vi "HandleIncomingPacket.vi"(8 "error in (no error)":errorcluster, 11 "ControlPacket in":refnum<class "ControlPacket.lvclass">) -> (0 "error out":errorcluster, 3 "ControlPacket out":refnum<class "ControlPacket.lvclass">)   [LabVIEW 2013, in "MQTT_Control_Packets.lvlib" / "ControlPacket.lvclass"]
uses:
  ControlPacket.lvclass
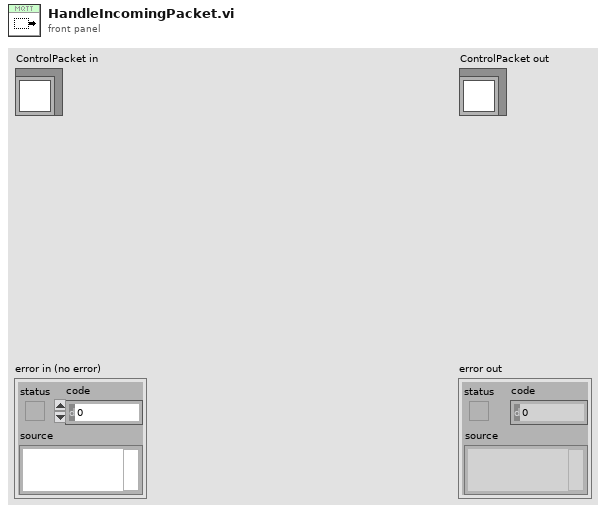
[diagram p1: front panel]
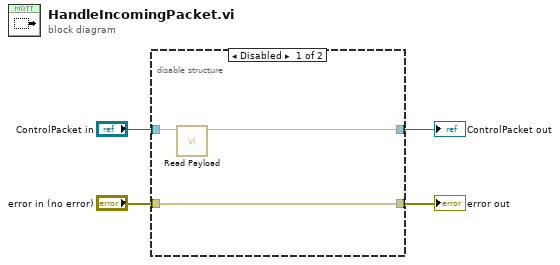
[diagram p0: block diagram]
diagram:
  n1 = disable-structure shown="Disabled" {
    disable-tunnel: "ControlPacket in" -> [w7 w8]
    disable-tunnel: [w6 w8] -> w3
    disable-tunnel: "error in (no error)" -> [w5 w9]
    disable-tunnel: [w5 w9] -> w1
    frame Disabled {
      n2 = call "Read Payload.vi"("ControlPacket in"=w7) -> ("ControlPacket out"=w6:refnum<class "ControlPacket.lvclass">)  [unwired: 9 in, 1 out]
    }
    frame Enabled {
    }
  }
  "error out" <- w1
  "ControlPacket out" <- w3
